vi "HTML Report Table Row.vi"(4 "vertical align (default)":T2, 5 "align (default)":T1, 6 "table cells":string, 7 "table rows in":string) -> (3 "table rows out":string)   [LabVIEW 2020, in "NI_ReportGenerationCore.lvlib"]
doc: "Constructs tags for an HTML table row <TR> with the specified row contents."
uses:
  NI_ReportGenerationCore.lvlib
  HTML Report Vertical Cell Alignment.ctl
  HTML Report Text Alignment.ctl
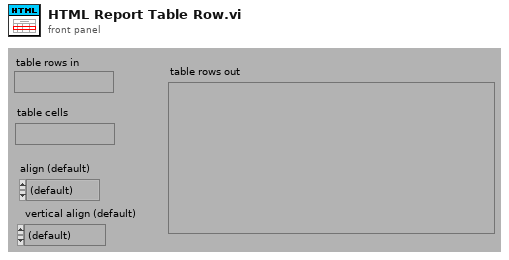
[diagram p1: front panel]
types:
  T1 = typedef "NI_ReportGenerationCore.lvlib/HTML Report Text Alignment.ctl" = enum16{"(default)", "LEFT", "CENTER", "RIGHT"}
  T2 = typedef "NI_ReportGenerationCore.lvlib/HTML Report Vertical Cell Alignment.ctl" = enum16{"(default)", "TOP", "MIDDLE", "BOTTOM"}
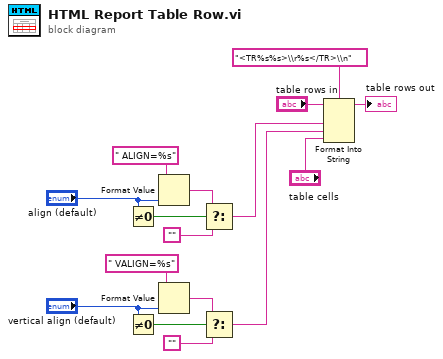
[diagram p0: block diagram]
diagram:
  n1 = Not Equal To 0?(x="align (default)") -> (x != 0?=w16:bool)
  n2 = Not Equal To 0?(x="vertical align (default)") -> (x != 0?=w8:bool)
  n3 = Format Value(format string=" ALIGN=%s", value (0)="align (default)") -> (output string=w15:string)  [unwired: 1 out]
  n4 = Format Value(format string=" VALIGN=%s", value (0)="vertical align (default)") -> (output string=w9:string)  [unwired: 1 out]
  n5 = Select(t=w15, s=w16, f="" ("Empty String Constant")) -> (s? t:f=w5:string)
  n6 = Select(t=w9, s=w8, f="" ("Empty String Constant")) -> (s? t:f=w4:string)
  n7 = Format Into String(format string="<TR%s%s>\\r%s</TR>\\n", initial string="table rows in", w5, w4, "table cells") -> (resulting string=→"table rows out":string)  [unwired: 1 in, 1 out]
